vi "Label_Prefix.vi"() -> (0 "Label Prefix String":string)   [LabVIEW 2016, in "Hardware.lvlib" / "Inclinometer.lvlib" / "Inclinometer Configuration.lvclass"]
uses:
  <userlib>/Common Components/Hardware/Inclinometer/Inclinometer Config/Inclinometer Configuration.lvclass
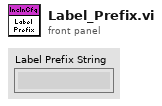
[diagram p1: front panel]
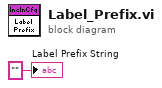
[diagram p0: block diagram]
diagram:
  "Label Prefix String" <- "" ("Label Prefix String")
